vi "Theta 0.vi"(10 "theta_6":dbl, 11 "6R Type 2 Serial Arm Class in":refnum<class "NI_Robotics_6R Type 2 Serial Arm Class.lvclass">) -> (2 "theta_0 array":dbl[](array[numeric]), 3 "6R Type 2 Serial Arm Class out":refnum<class "NI_Robotics_6R Type 2 Serial Arm Class.lvclass">)   [LabVIEW 2017, in "NI_Robotics_6R Type 2 Serial Arm Class.lvclass"]
uses:
  <vilib>/robotics/Kinematics/Analytical/6R/Type 2/NI_Robotics_6R Type 2 Serial Arm Class.lvclass
  c:/Program Files (x86)/National Instruments/LabVIEW 2017/vi.lib/robotics/Kinematics/Analytical/Generic/NI_Robotics_Analytical Serial Arm Class.lvclass
  <vilib>/robotics/Kinematics/Link/NI_Robotics_Link.lvclass/NI_Robotics_Link.ctl
  <vilib>/robotics/Kinematics/Link/Get Kinematic Parameters.vi
  <vilib>/robotics/Kinematics/Analytical/Generic/NI_Robotics_Analytical Serial Arm Class.lvclass
  c:/Program Files (x86)/National Instruments/LabVIEW 2017/vi.lib/robotics/Kinematics/Robot/NI_Robotics_Serial Robot Arm.lvclass
  <vilib>/robotics/Kinematics/Analytical/Generic/Accessors/Read alpha_n0.vi
  <vilib>/robotics/Kinematics/Robot/Get Links.vi
panel:
  out "output variable 2":dbl
  out "output variable":dbl
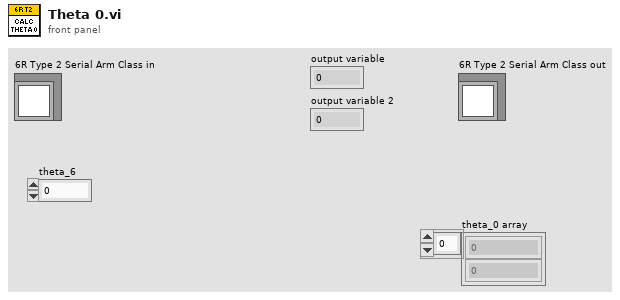
[diagram p1: front panel]
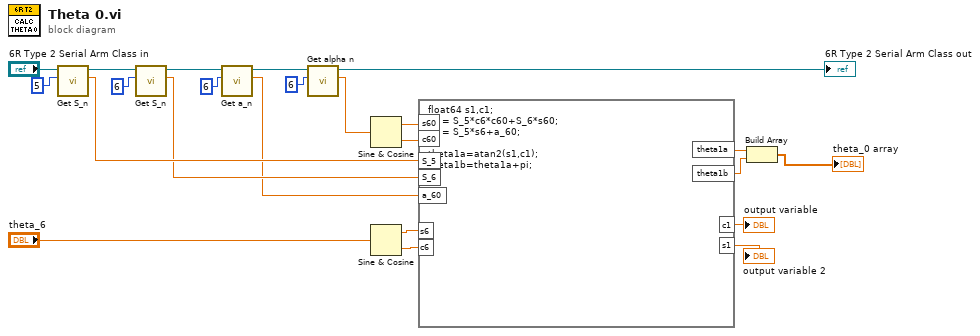
[diagram p0: block diagram]
diagram:
  n1 = call <vilib>:"Get S_n.vi"("n"=5, "Analytical Serial Arm Class in"="6R Type 2 Serial Arm Class in") -> ("S_n"=w8:dbl, "Analytical Serial Arm Class out"=w19:refnum<class "NI_Robotics_6R Type 2 Serial Arm Class.lvclass">)  [unwired: 8 in]
  n2 = call <vilib>:"Get S_n.vi"("n"=6, "Analytical Serial Arm Class in"=w19) -> ("S_n"=w7:dbl, "Analytical Serial Arm Class out"=w17:refnum<class "NI_Robotics_6R Type 2 Serial Arm Class.lvclass">)  [unwired: 8 in]
  n3 = call <vilib>:"Get a_n.vi"("n"=6, "Analytical Serial Arm Class in"=w17) -> ("a_n"=w6:dbl, "Analytical Serial Arm Class out"=w15:refnum<class "NI_Robotics_6R Type 2 Serial Arm Class.lvclass">)  [unwired: 8 in]
  n4 = call <vilib>:"Get alpha n.vi"("n"=6, "Analytical Serial Arm Class in"=w15) -> ("alpha n"=w13:dbl, "Analytical Serial Arm Class out"=→"6R Type 2 Serial Arm Class out":refnum<class "NI_Robotics_6R Type 2 Serial Arm Class.lvclass">)  [unwired: 8 in]
  n5 = Sine & Cosine(0:w13) -> (1:w12:dbl, 2:w11:dbl)
  n6 = Sine & Cosine(0:"theta_6") -> (1:w9:dbl, 2:w10:dbl)
  n7 = formula code="float64 s1,c1;\ns1 = S_5*c6*c60+S_6*s60;\nc1 = S_5*s6+a_60;\n\ntheta1a=atan2(s1,c1);\ntheta1b=theta1a+pi;"("c60"=w11, "s60"=w12, "s6"=w9, "c6"=w10, "S_5"=w8, "S_6"=w7, "a_60"=w6) -> ("theta1a"=w5:dbl, "theta1b"=w4:dbl, "c1"=→"output variable":dbl, "s1"=→"output variable 2":dbl)
  n8 = Build Array(w5, w4) -> (→"theta_0 array":dbl[])
